vi "rotation_control.vi"(4 "Continuous output":bool, 6 "Wait for completion?":bool=TRUE, 7 "Triggered start?":bool, 8 "Rotation orientation":bool, 9 "waiting time":dbl=0.01 format="%#_13p", 10 "Duration of rotation":dbl, 11 "Number of pulses":i32=100) -> (0 "task out":refnum<k21>, 3 "pulse duration (T/2)":dbl=0.001 format="%#_13p")   [LabVIEW 2019]
uses:
  <vilib>/DAQmx/write.llb/DAQmx Write (Digital 1D Wfm NChan NSamp).vi
  global_variables.vi
  <vilib>/Waveform/DWDTOps.llb/DWDT Digital Size.vi
  <vilib>/DAQmx/create/channels.llb/DAQmx Create Channel (DO-Digital Output).vi
  <vilib>/DAQmx/configure/timing.llb/DAQmx Timing (Sample Clock).vi
  <vilib>/Waveform/DWDTOps.llb/DWDT Uncompress Digital.vi
  <vilib>/DAQmx/miscellaneous.llb/DAQmx Fill In Error Info.vi
  <vilib>/DAQmx/configure/trigger.llb/DAQmx Start Trigger (Digital Edge).vi
panel:
  out "?":bool
  out "number of samples":i32
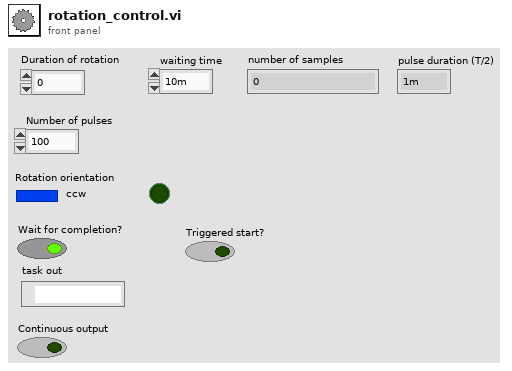
[diagram p1: front panel]
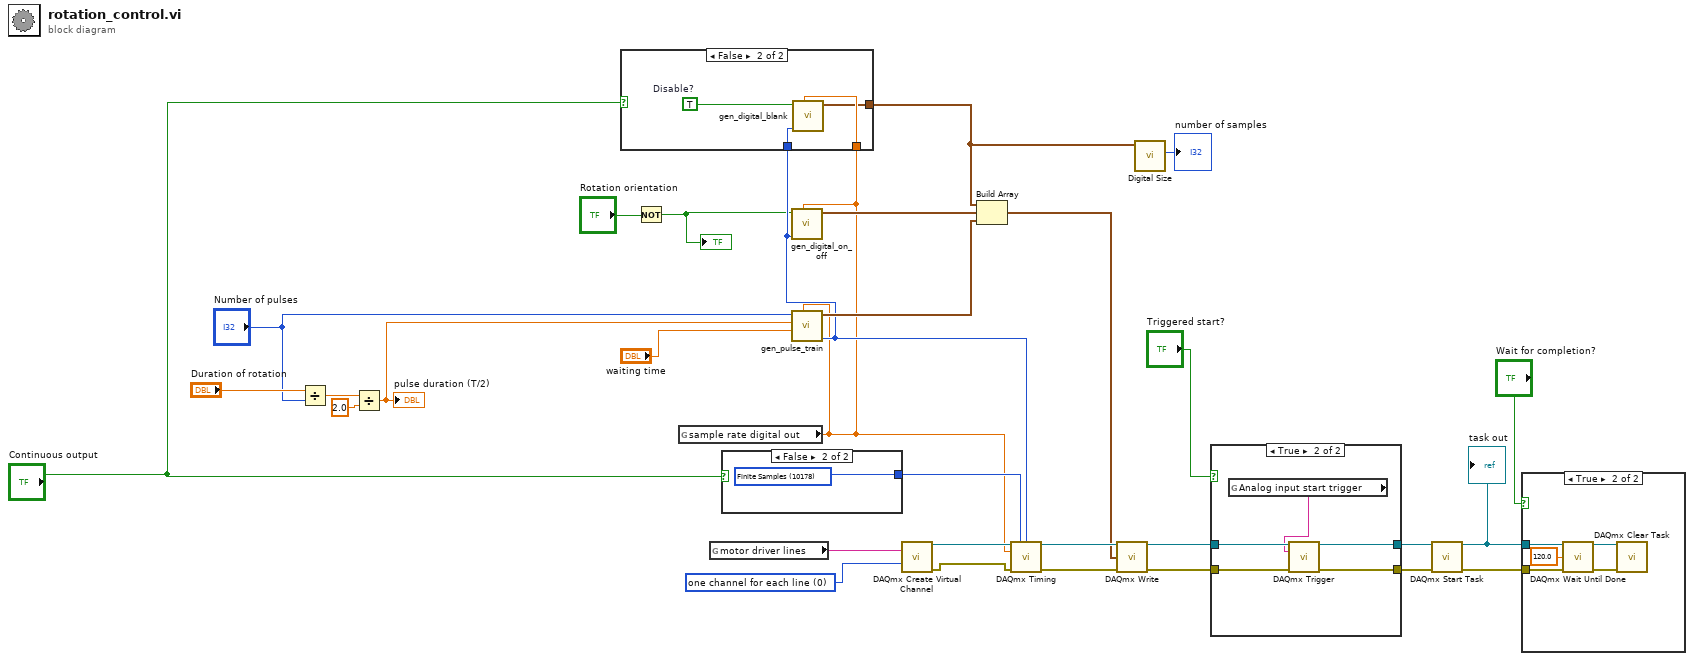
[diagram p0: block diagram]
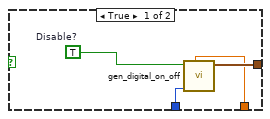
[diagram p2: hidden frame]
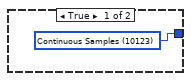
[diagram p3: hidden frame]
diagram:
  w23 = 0 items=["one channel for each line", "one channel for all lines"] ("line grouping")
  n1 = Divide(x="Duration of rotation", y="Number of pulses") -> (x/y=w6:dbl)
  n2 = Divide(x=w6, y=2.0) -> (x/y=w4:dbl)
  "pulse duration (T/2)" <- w4
  n3 = Not(x="Rotation orientation") -> (.not. x?=w2:bool)
  "?" <- w2
  n4 = global read "global_variables.vi" "sample rate digital out"() -> (w18:dbl)
  n5 = global read "global_variables.vi" "motor driver lines"() -> (w1:tag)
  n6 = case shown="False" "Continuous output" {
    tunnel: [w32 w33] -> w29
    frame True {
      w32 = 10123 items=["Finite Samples"=10178, "Continuous Samples"=10123, "Hardware Timed Single Point"=12522] ("sample mode")
    }
    frame False {
      w33 = 10178 items=["Finite Samples"=10178, "Continuous Samples"=10123, "Hardware Timed Single Point"=12522] ("sample mode")
    }
  }
  n7 = call "gen_pulse_train.vi"("sampling rate"=w18, "waiting time"="waiting time", "pulse width"=w4, "Number of pulses"="Number of pulses") -> ("waveform length"=w20:i32, "digital waveform out"=w22:digitalwaveform)  [unwired: 6 in]
  n8 = case shown="False" "Continuous output" {
    tunnel: w20 -> [w36 w41]
    tunnel: w18 -> [w35 w39]
    tunnel: [w37 w38] -> w11
    frame True {
      w34 = TRUE  # Disable?
      n9 = call "gen_digital_on_off.vi"("sampling rate"=w35, "waveform length"=w36, "On / Off"=w34) -> ("digital waveform"=w37:digitalwaveform)  [unwired: 8 in]
    }
    frame False {
      w40 = TRUE  # Disable?
      n10 = call "gen_digital_blank.vi"("sampling rate"=w39, "waveform length"=w41, "On / Off"=w40) -> ("digital waveform"=w38:digitalwaveform)  [unwired: 8 in]
    }
  }
  n11 = call "gen_digital_on_off.vi"("sampling rate"=w18, "waveform length"=w20, "On / Off"=w2) -> ("digital waveform"=w21:digitalwaveform)  [unwired: 8 in]
  n12 = call-poly <vilib>:"DAQmx Create Virtual Channel.vi"("lines"=w1, "line grouping"=w23) -> ("task out"=w30:refnum<k21>, "error out"=w26:errorcluster)  [unwired: 12 in]
  n13 = Build Array(w11, w21, w22) -> (w19:digitalwaveform[])
  n14 = call-poly <vilib>:"DAQmx Timing.vi"("task/channels in"=w30, "sample mode"=w29, "samples per channel"=w20, "rate"=w18, "error in"=w26) -> ("task out"=w28:refnum<k21>, "error out"=w27:errorcluster)  [unwired: 9 in]
  n15 = call-poly <vilib>:"DAQmx Write.vi"("task/channels in"=w28, "data"=w19, "error in"=w27) -> ("task out"=w16:refnum<k21>, "error out"=w15:errorcluster)  [unwired: 10 in, 1 out]
  n16 = call-poly <vilib>:"Digital Size.vi"("digital waveform in"=w11) -> ("number of samples"=→"number of samples":i32)  [unwired: 7 in, 3 out]
  n17 = case shown="True" "Triggered start?" {
    tunnel: w16 -> [w43 w48]
    tunnel: w15 -> [w42 w47]
    tunnel: [w43 w46] -> w14
    tunnel: [w42 w45] -> w13
    frame False {
    }
    frame True {
      n18 = global read "global_variables.vi" "Analog input start trigger"() -> (w44:tag)
      n19 = call-poly <vilib>:"DAQmx Trigger.vi"("task/channels in"=w48, "source"=w44, "error in"=w47) -> ("task out"=w46:refnum<k21>, "error out"=w45:errorcluster)  [unwired: 11 in]
    }
  }
  n20 = call <vilib>:"DAQmx Start Task.vi"("task/channels in"=w14, "error in"=w13) -> ("task out"=w25:refnum<k21>, "error out"=w24:errorcluster)  [unwired: 12 in]
  "task out" <- w25
  n21 = case shown="True" "Wait for completion?" {
    tunnel: w25 -> [_ w53]
    tunnel: w24 -> [_ w52]
    frame False {
    }
    frame True {
      n22 = call <vilib>:"DAQmx Wait Until Done.vi"("task/channels in"=w53, "timeout (sec)"=120.0, "error in"=w52) -> ("task out"=w50:refnum<k21>, "error out"=w51:errorcluster)  [unwired: 11 in]
      n23 = call <vilib>:"DAQmx Clear Task.vi"("task in"=w50, "error in"=w51) -> ()  [unwired: 13 in, 1 out]
    }
  }
